vi "arrays.vi"() -> ()   [LabVIEW 2018]
panel:
  out "Index indicator":dbl
  out "Array size":dbl
  out "Array indicator":dbl[](array[slide]) scale=0.0..10.0
  in  "Array control":dbl[](array[numeric])
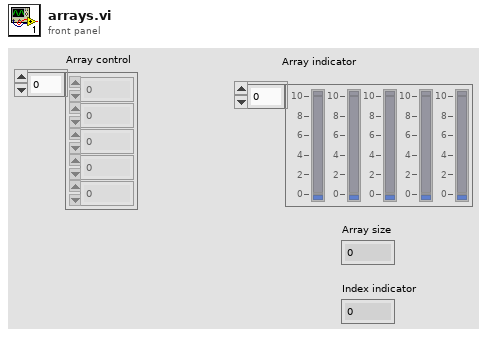
[diagram p1: front panel]
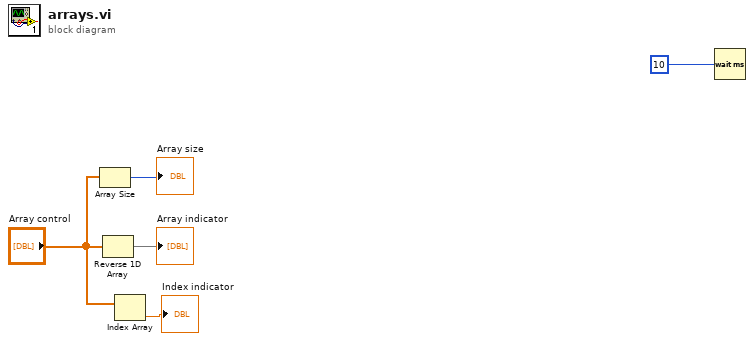
[diagram p0: block diagram]
diagram:
  n1 = Array Size(array="Array control") -> (size(s)=→"Array size":i32)
  n2 = Reverse 1D Array(array="Array control") -> (reversed array=→"Array indicator":dbl[])
  n3 = Index Array(array="Array control") -> (element=→"Index indicator":dbl)  [unwired: 1 in]
  n4 = Wait (ms)(milliseconds to wait=10) -> ()  [unwired: 1 out]
